vi "Mod_OFDM_Set_Ofdm_Symbol_Pool.vi"(0 "Configuration out":variant, 7 "Current OFDM \nSymbol NAME":string, 11 "error in":errorcluster) -> (4 "Configuration out":variant=variant("OFDM SYMBOL POOL"=variant(string[] ["ABC", "AWER", ""])), 8 "index of current Symbol":i32=2, 10 "OFDM Symbol pool":string[](array[string])=["ABC", "AWER", ""], 15 "error out":errorcluster)   [LabVIEW 2010]
uses:
  MOD_OFDM_Get_Attr.vi
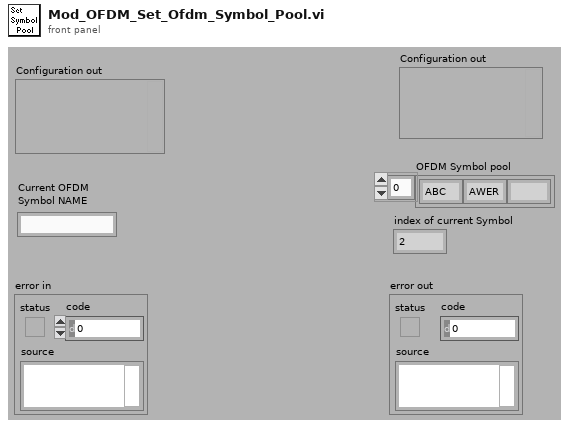
[diagram p1: front panel]
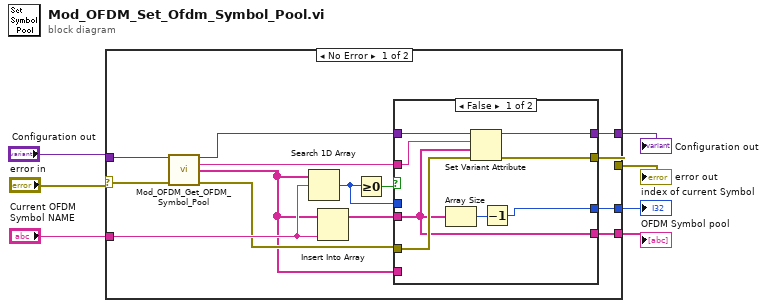
[diagram p0: block diagram]
diagram:
  n1 = case shown="No Error" "error in" {
    selector: "error in" -> [w8 w34]
    tunnel: "Current OFDM \nSymbol NAME" -> [w19 _]
    tunnel: [w18 _] -> w6
    tunnel: [w17 w34] -> w5
    tunnel: [w16 _] -> w4
    tunnel: "Configuration out" -> [w15 _]
    tunnel: [w13 _] -> w2
    frame No Error {
      n2 = call-poly "Mod_OFDM_Get_OFDM_Symbol_Pool.vi"("Configuration in"=w15, "error in"=w8) -> ("Configuration out"=w10:variant, "Attribute Name"=w9:string, "Symbol Pool"=w11:string[], "error out"=w12:errorcluster)  [unwired: 8 in, 2 out]
      n3 = Search 1D Array(1D array=w11, element=w19) -> (index of element=w14:i32)  [unwired: 1 in]
      n4 = Insert Into Array(array=w11, new element=w19) -> (w20:string[])  [unwired: 1 in]
      n5 = Greater Or Equal To 0?(x=w14) -> (x >= 0?=w21:bool)
      n6 = case shown="False" w21 {
        tunnel: w20 -> [w24 _]
        tunnel: w10 -> [w29 w33]
        tunnel: [w27 w33] -> w18
        tunnel: w9 -> [w28 _]
        tunnel: w12 -> [w26 w32]
        tunnel: [w25 w32] -> w17
        tunnel: w11 -> [_ w31]
        tunnel: [w24 w31] -> w16
        tunnel: w14 -> [_ w30]
        tunnel: [w22 w30] -> w13
        frame False {
          n7 = Array Size(array=w24) -> (size(s)=w23:i32)
          n8 = Set Variant Attribute(Variant=w29, name=w28, value=w24, error in=w26) -> (Variant out=w27:variant, error out=w25:errorcluster)  [unwired: 1 out]
          n9 = Decrement(x=w23) -> (x-1=w22:i32)
        }
        frame True {
        }
      }
    }
    frame Error {
    }
  }
  "Configuration out" <- w6
  "error out" <- w5
  "OFDM Symbol pool" <- w4
  "index of current Symbol" <- w2
